vi "Config_Graph Out.vi"(10 "Graph Cluster 3":T1, 11 "Graph Cluster in":T2) -> (3 "Graph Cluster out":T2)   [LabVIEW 2012]
doc: "This .vi configures the graphs to be displayed in Graph Cluster Out."
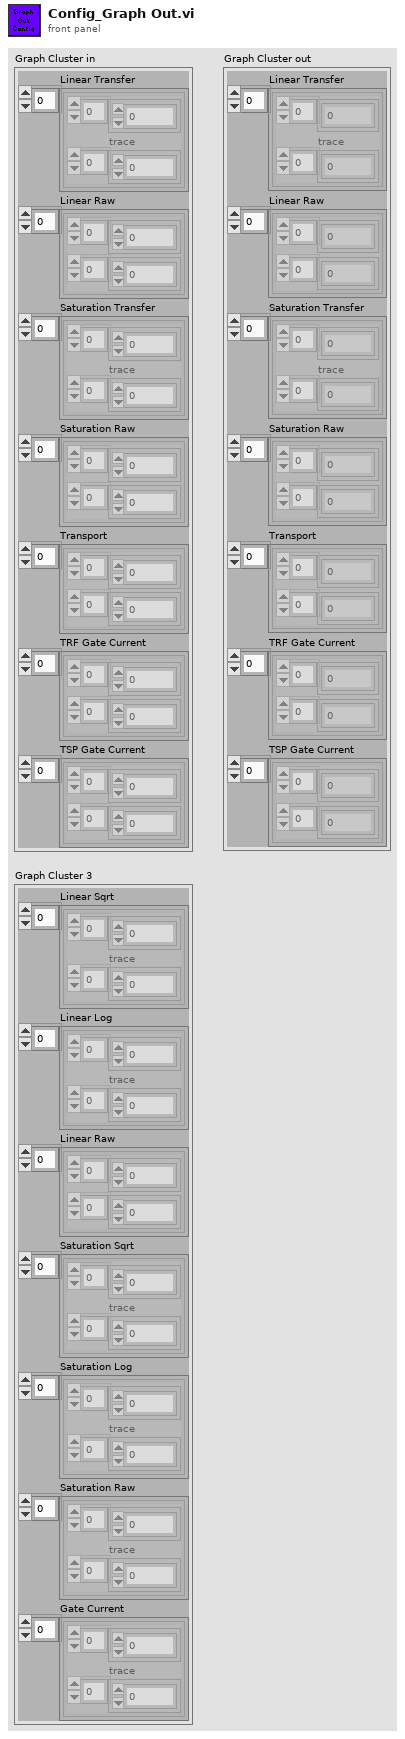
[diagram p1: front panel]
types:
  T1 = cluster{"Linear Sqrt":cluster{dbl[], "trace":dbl[]}[], "Linear Log":cluster{dbl[], "trace":dbl[]}[], "Linear Raw":cluster{dbl[], dbl[]}[], "Saturation Sqrt":cluster{dbl[], "trace":dbl[]}[], "Saturation Log":cluster{dbl[], "trace":dbl[]}[], "Saturation Raw":cluster{dbl[], "trace":dbl[]}[], "Gate Current":cluster{dbl[], "trace":dbl[]}[]}
  T2 = cluster{"Linear Transfer":cluster{dbl[], "trace":dbl[]}[], "Linear Raw":cluster{dbl[], dbl[]}[], "Saturation Transfer":cluster{dbl[], "trace":dbl[]}[], "Saturation Raw":cluster{dbl[], dbl[]}[], "Transport":cluster{dbl[], dbl[]}[], "TRF Gate Current":cluster{dbl[], dbl[]}[], "TSP Gate Current":cluster{dbl[], dbl[]}[]}
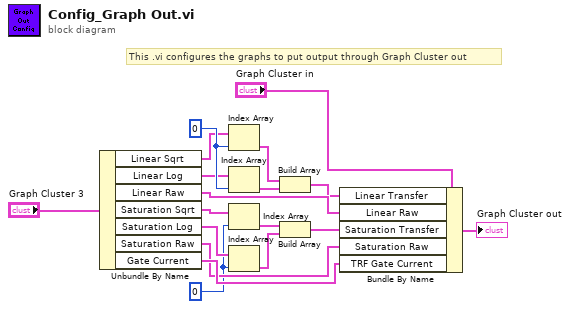
[diagram p0: block diagram]
diagram:
  w11 = 0
  w5 = 0
  # "This .vi configures the graphs to put output through Graph Cluster out"
  n1 = Unbundle By Name("Graph Cluster 3") -> ("Linear Sqrt"=w3:cluster{dbl[], "trace":dbl[]}[], "Linear Log"=w4:cluster{dbl[], "trace":dbl[]}[], "Linear Raw"=w15:cluster{dbl[], dbl[]}[], "Saturation Sqrt"=w12:cluster{dbl[], "trace":dbl[]}[], "Saturation Log"=w13:cluster{dbl[], "trace":dbl[]}[], "Saturation Raw"=w16:cluster{dbl[], "trace":dbl[]}[], "Gate Current"=w18:cluster{dbl[], "trace":dbl[]}[])
  n2 = Index Array(array=w3, index=w5) -> (element=w6:cluster{dbl[], "trace":dbl[]})
  n3 = Index Array(array=w4, index=w5) -> (element=w7:cluster{dbl[], "trace":dbl[]})
  n4 = Index Array(array=w12, index=w11) -> (element=w10:cluster{dbl[], "trace":dbl[]})
  n5 = Index Array(array=w13, index=w11) -> (element=w9:cluster{dbl[], "trace":dbl[]})
  n6 = Build Array(w6, w7) -> (w8:cluster{dbl[], "trace":dbl[]}[])
  n7 = Build Array(w10, w9) -> (w14:cluster{dbl[], "trace":dbl[]}[])
  n8 = Bundle By Name(cluster="Graph Cluster in", "Linear Transfer"=w8, "Linear Raw"=w15, "Saturation Transfer"=w14, "Saturation Raw"=w16, "TRF Gate Current"=w18) -> (→"Graph Cluster out":T2)
